vi "Draw Block.vi"(9 "State":T1, 11 "Picture In":picture) -> (3 "Picture":picture)   [LabVIEW 2020, in "Parallel Diagram Block.xnode"]
uses:
  Parallel Diagram Block.xnode
  <vilib>/XNodeSupport/XNodeInt.ctl
  <vilib>/XNodeSupport/NI_XNodeSupport.lvlib
  Parallel Block/Value Type.ctl
  Parallel Block/Parallel Block.lvlib
  Parallel Block/Type Descriptor.ctl
  <vilib>/picture/picture.llb/imagedata.ctl
  Parallel Block/Direction.ctl
  Parallel Block/IO Selection.ctl
  State.ctl
  Parallel Block/Terminal Mode.ctl
  Parallel Block/Terminal Type.ctl
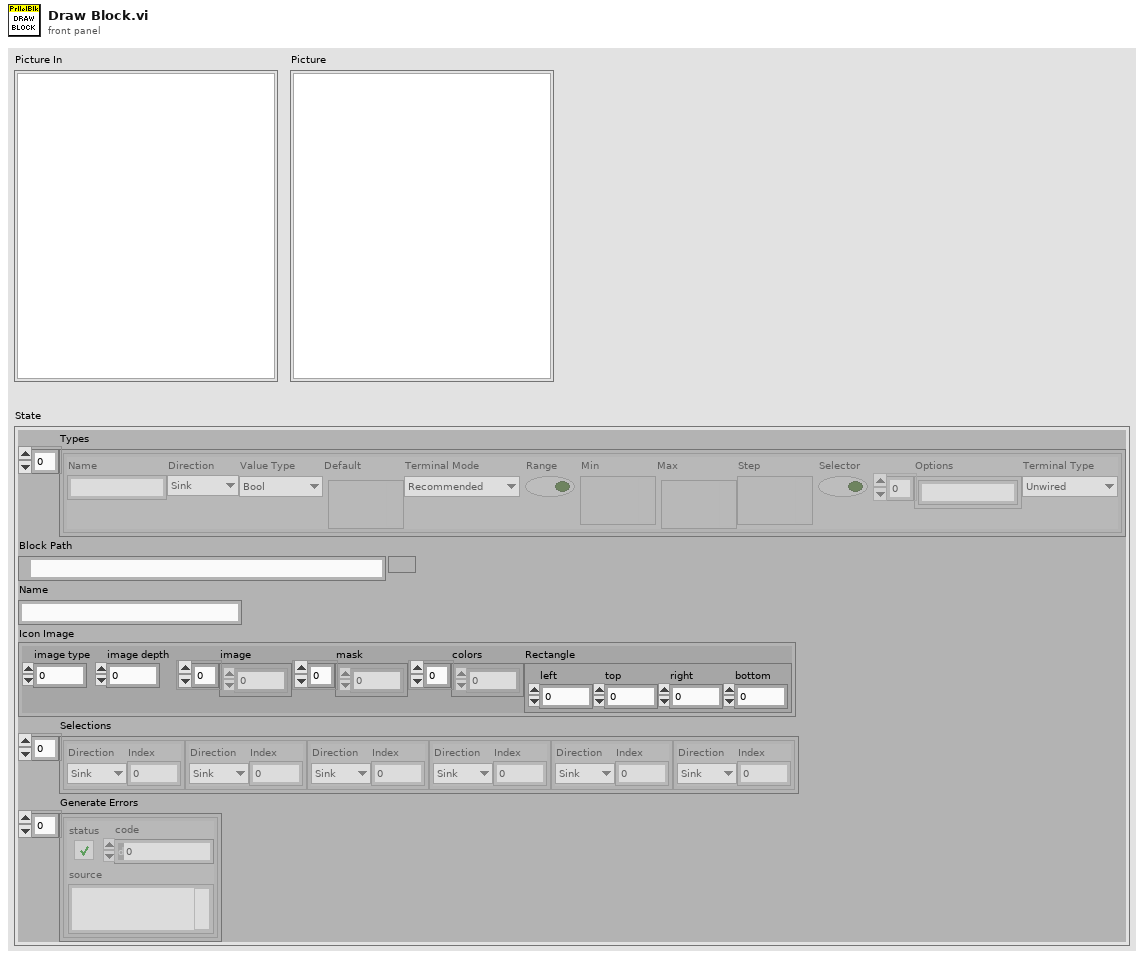
[diagram p1: front panel]
types:
  T1 = typedef "Parallel Diagram Block.xnode/State.ctl" = cluster{"Types":T2[], "Block Path":path, "Name":string, "Icon Image":T7, "Selections":T8[], "Generate Errors":errorcluster[]}
  T2 = typedef "Parallel Block.lvlib/Type Descriptor.ctl" = cluster{"Name":string, "Direction":T3, "Value Type":T4, "Default":variant, "Terminal Mode":T5, "Range":bool, "Min":variant, "Max":variant, "Step":variant, "Selector":bool, "Options":string[], "Terminal Type":T6}
  T3 = typedef "Parallel Block.lvlib/Direction.ctl" = enum16{"Sink", "Source"}
  T4 = typedef "Parallel Block.lvlib/Value Type.ctl" = enum16{"Unknown", "Bool", "U8", "U16", "U32", "U64", "I8", "I16", "I32", "I64", "SGL", "DBL", "CSG", "CDB", "CDBWfm", "String", "DBLWfm"}
  T5 = typedef "Parallel Block.lvlib/Terminal Mode.ctl" = enum16{"Recommended", "Required", "None"}
  T6 = typedef "Parallel Block.lvlib/Terminal Type.ctl" = enum16{"Unwired", "Connection", "Value", "Control Ref"}
  T7 = typedef "imagedata.ctl" = cluster{"image type":i32, "image depth":i32, "image":u8[], "mask":u8[], "colors":u32[], "Rectangle":cluster{"left":i16, "top":i16, "right":i16, "bottom":i16}}
  T8 = typedef "Parallel Block.lvlib/IO Selection.ctl" = cluster{"Direction":T3, "Index":i32}
  T9 = cluster{"left":i16, "top":i16, "right":i16, "bottom":i16}
  T10 = typedef "NI_XNodeSupport.lvlib/XNodeInt.ctl" = i32
  T11 = cluster{"horizontal":enum16{"left", "center", "right"}, "vertical":enum16{"top", "center", "bottom"}}
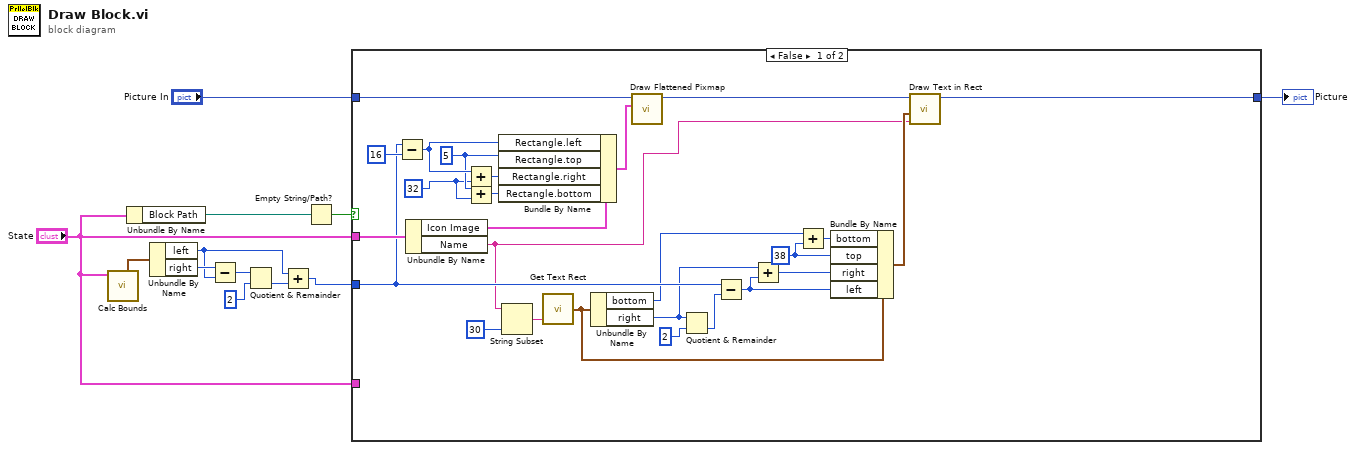
[diagram p0: block diagram]
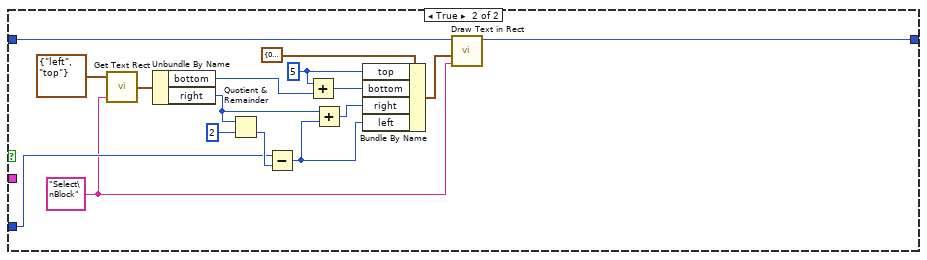
[diagram p2: hidden frame]
diagram:
  n1 = call "Calc Bounds.vi"("State"="State") -> ("Border Without Terminals"=w7:T9)  [unwired: 7 in, 3 out]
  n2 = Unbundle By Name("State") -> ("Block Path"=w9:path)
  n3 = Unbundle By Name(w7) -> ("left"=w3:i16, "right"=w6:i16)
  n4 = Subtract(x=w6, y=w3) -> (x-y=w5:i16)
  n5 = Quotient & Remainder(x=w5, y=2) -> (floor(x/y)=w4:i32)  [unwired: 1 out]
  n6 = Add(x=w3, y=w4) -> (x+y=w2:i32)
  n7 = Empty String/Path?(string/path=w9) -> (empty?=w8:bool)
  n8 = case shown="False" w8 {
    tunnel: "Picture In" -> [w38 w53]
    tunnel: "State" -> [w30 _]
    tunnel: [w13 w39] -> w11
    tunnel: w2 -> [w24 w41]
    tunnel: "State" -> [_ _]
    frame False {
      w16 = i16 38 ("top")
      w32 = T10 32 ("y")
      w35 = i16 5 ("Rectangle.top")
      n9 = Subtract(x=w24, y=T10 16) -> (x-y=w37:T10)
      n10 = Unbundle By Name(w30) -> ("Icon Image"=w29:T7, "Name"=w14:string)
      n11 = Add(x=w37, y=w32) -> (x+y=w36:T10)
      n12 = Add(x=w35, y=w32) -> (x+y=w34:T10)
      n13 = Bundle By Name(cluster=w29, "Rectangle.left"=w37, "Rectangle.top"=w35, "Rectangle.right"=w36, "Rectangle.bottom"=w34) -> (w31:T7)
      n14 = String Subset(string=w14, length (rest)=30 ("length (rest)")) -> (substring=w27:string)  [unwired: 1 in]
      n15 = call <vilib>:"Get Text Rect.vi"("text"=w27) -> ("rect"=w22:T9)  [unwired: 8 in]
      n16 = Unbundle By Name(w22) -> ("bottom"=w15:i16, "right"=w19:i16)
      n17 = call <vilib>:"Draw Flattened Pixmap.vi"("image data"=w31, "picture"=w38) -> ("new picture"=w25:picture)  [unwired: 7 in]
      n18 = Quotient & Remainder(x=w19, y=i16 2) -> (floor(x/y)=w23:i16)  [unwired: 1 out]
      n19 = Subtract(x=w24, y=w23) -> (x-y=w20:i32)
      n20 = Add(x=w19, y=w20) -> (x+y=w21:i32)
      n21 = Add(x=w15, y=w16) -> (x+y=w17:i16)
      n22 = Bundle By Name(cluster=w22, "bottom"=w17, "top"=w16, "right"=w21, "left"=w20) -> (w18:T9)
      n23 = call <vilib>:"Draw Text in Rect.vi"("text"=w14, "rect"=w18, "picture"=w25) -> ("new picture"=w13:picture)  [unwired: 8 in]
    }
    frame True {
      w47 = i16 5 ("top")
      w40 = "Select\nBlock" ("text")
      n24 = call <vilib>:"Get Text Rect.vi"("alignment(left, top)"=T11 {"horizontal"=enum."left", "vertical"=enum."top"}, "text"=w40) -> ("rect"=w52:T9)  [unwired: 7 in]
      n25 = Unbundle By Name(w52) -> ("bottom"=w46:i16, "right"=w43:i16)
      n26 = Quotient & Remainder(x=w43, y=i16 2) -> (floor(x/y)=w51:i16)  [unwired: 1 out]
      n27 = Subtract(x=w41, y=w51) -> (x-y=w44:i32)
      n28 = Add(x=w47, y=w46) -> (x+y=w48:i16)
      n29 = Add(x=w43, y=w44) -> (x+y=w45:i32)
      n30 = Bundle By Name(cluster=T9 {"left"=0, "top"=0, "right"=0, "bottom"=0} ("rect"), "top"=w47, "bottom"=w48, "right"=w45, "left"=w44) -> (w49:T9)
      n31 = call <vilib>:"Draw Text in Rect.vi"("text"=w40, "rect"=w49, "picture"=w53) -> ("new picture"=w39:picture)  [unwired: 8 in]
    }
  }
  "Picture" <- w11
